vi "Untitled 4 (SubVI) 1.vi"(6 "alignment correction":dbl, 7 "background \n coincidence counts":dbl, 9 "Array":ext[](array[numeric]), 10 "Numeric":ext, 11 "Array 2":ext[](array[numeric])) -> (3 "Cluster":cluster{ext[], ext[]})   [LabVIEW 2013]
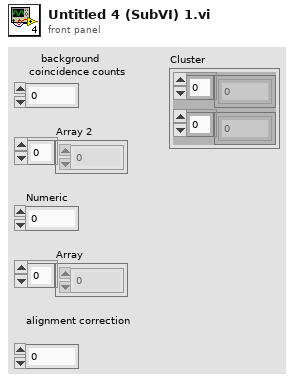
[diagram p1: front panel]
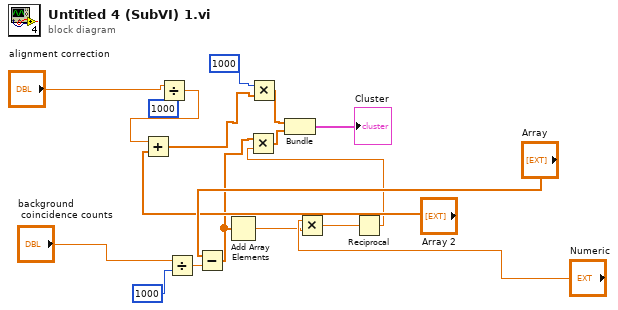
[diagram p0: block diagram]
diagram:
  n1 = Divide(x="alignment correction", y=1000) -> (x/y=w2:dbl)
  n2 = Add(x=w2, y="Array 2") -> (x+y=w16:ext[])
  n3 = Divide(x="background \n coincidence counts", y=1000) -> (x/y=w4:dbl)
  n4 = Subtract(x="Array", y=w4) -> (x-y=w8:ext[])
  n5 = Add Array Elements(numeric array=w8) -> (sum=w9:ext)
  n6 = Multiply(x=1000, y=w16) -> (x*y=w15:ext[])
  n7 = Multiply(x="Numeric", y=w9) -> (x*y=w10:ext)
  n8 = Reciprocal(x=w10) -> (1/x=w11:ext)
  n9 = Multiply(x=w8, y=w11) -> (x*y=w7:ext[])
  n10 = Bundle(w15, w7) -> (→"Cluster":cluster{ext[], ext[]})  [unwired: 1 in]
